vi "Obtain Groups.vi"(8 "error in (no error)":errorcluster, 11 "GenericGuiAI in":refnum<class "GenericGuiAI.lvclass">) -> (0 "error out":errorcluster, 3 "GenericGuiAI out":refnum<class "GenericGuiAI.lvclass">)   [LabVIEW 2020, in "VolatusDAQGenericGUI.lvlib" / "GenericGuiAI.lvclass"]
uses:
  GenericGuiAI.lvclass
  C:/dev/lv20CE/relink/lv-volatus/Volatus/Module/Module.lvclass
  Volatus/Module/Module.lvclass/Module.ctl
  GenericGuiAI.lvclass/GenericGuiAI.ctl
  VolatusConfig/VolatusConfigElement/VolatusConfigElement.lvclass/VolatusConfigElement.ctl
  VolatusConfig/VolatusConfigElement/Element.vi
  VolatusConfig/Group/Group.lvclass
  C:/dev/lv20CE/relink/lv-volatus/VolatusConfig/VolatusConfigElement/VolatusConfigElement.lvclass
  lv-cdm/CDM-Config/Config Element/Name.vi
  Volatus/Module/Module.lvclass
  VolatusDAQGenericGUI.lvlib
  C:/dev/lv20CE/relink/lv-volatus/VolatusDAQGenericGUI/GenericGuiAI/GenericGuiAI.lvclass
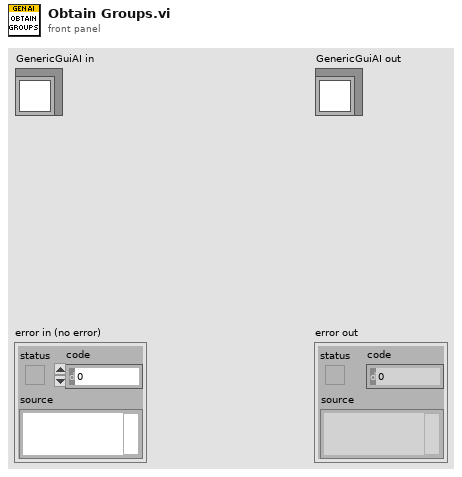
[diagram p1: front panel]
types:
  T1 = typedef "VolatusDAQGenericGUI.lvlib/Group Info.ctl" = cluster{"Group":refnum<class "Group.lvclass">, "Channel Names":string[], "Resources":string[], "Node":string, "Task":string}
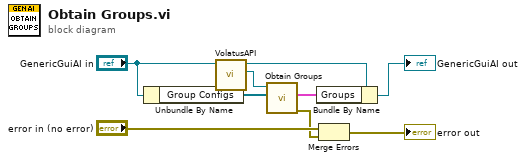
[diagram p0: block diagram]
diagram:
  n1 = Unbundle By Name("GenericGuiAI in") -> ("Group Configs"=w4:refnum<class "Group.lvclass">[])
  n2 = call "VolatusAPI.vi"("Module in"="GenericGuiAI in") -> ("VolatusAPI"=w3:refnum<class "VolatusAPI.lvclass">, "Module out"=w8:refnum<class "GenericGuiAI.lvclass">)  [unwired: 9 in]
  n3 = call "Obtain Groups.vi"("Group Configs"=w4, "VolatusAPI"=w3) -> ("error out"=w1:errorcluster, "Groups"=w2:T1[])  [unwired: 8 in]
  n4 = Bundle By Name(cluster=w8, "Groups"=w2) -> (→"GenericGuiAI out":refnum<class "GenericGuiAI.lvclass">)
  n5 = Merge Errors("error in (no error)", w1) -> (→"error out":errorcluster)
